vi "Highlight Selected Row in Table Control 2012 NIVerified.vi"() -> ()   [LabVIEW 2012]
doc: "This example lets you highlight a row based on which row a user clicks on. It changes the background color and then changes it back to blank when another row is clicked on."
panel:
  in  "stop":bool
  in  "Table Control":string[][](table)
  # "Overview: This example demonstrates a common practice of dealing with Tables programmatically,which lets you highlight a row based on which row a user clicks on. \nRequirements: LabVIEW 2012 (or compatible)\nInstruction:\n1. Run the VI\n2. Click on a row to highlight it."
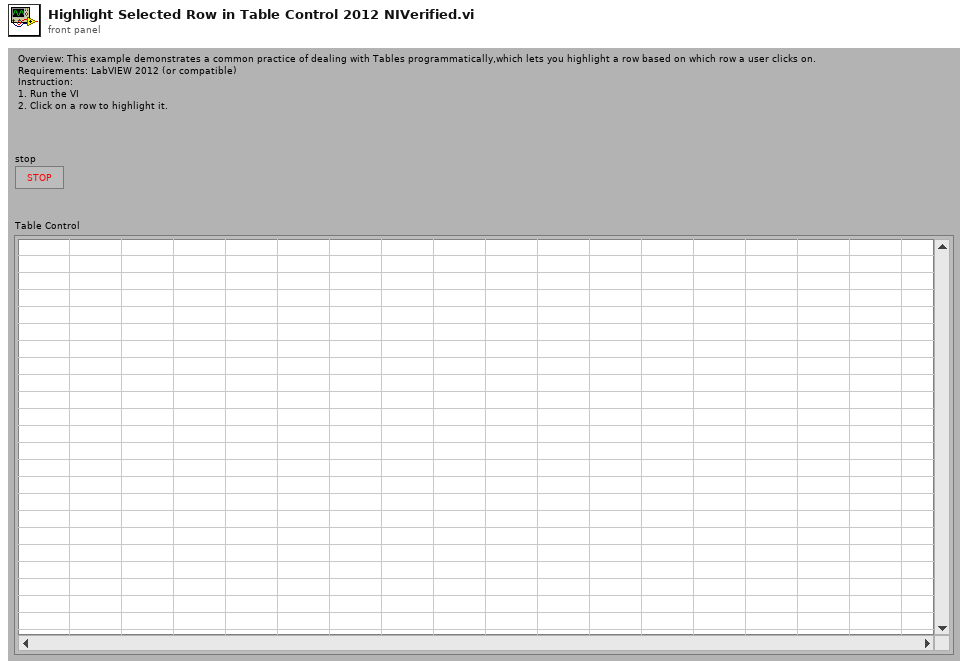
[diagram p1: front panel]
types:
  T1 = typedef "LVRowAndColumnTypeDef.ctl" = cluster{"Row":i32, "Column":i32}
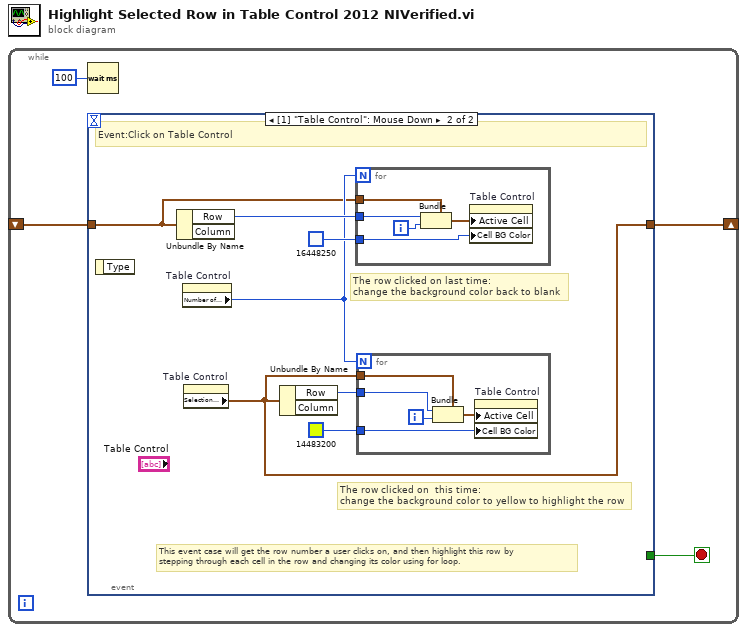
[diagram p0: block diagram]
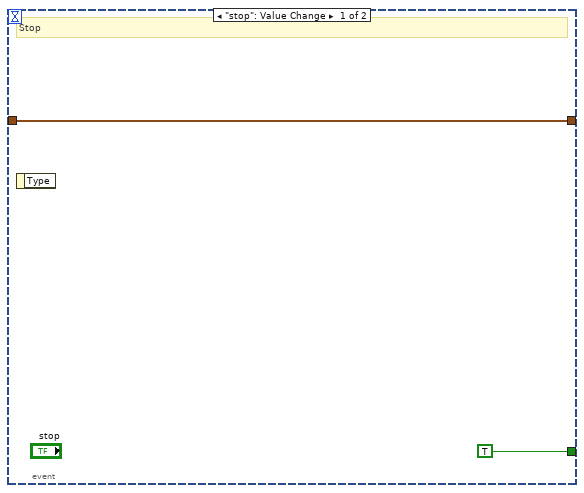
[diagram p2: hidden frame]
diagram:
  n1 = while {
    shift-right: [w3] -> _
    shift-left: _ -> [w2]
    stop <- w1 stop-if-true
    n2 = Wait (ms)(milliseconds to wait=u32 100) -> ()  [unwired: 1 out]
    n3 = event shown="[1] \"Table Control\": Mouse Down" {
      selector: _ -> [_ _]
      dyn-events: _ -> [_ _]
      timeout: _ -> [_ _]
      tunnel: [w6 w7] -> w3
      tunnel: w2 -> [w6 w8]
      tunnel: [TRUE _] -> w1
      event "stop": Value Change {
        # "Stop"
        n4 = event-data() -> ()  [unwired: 1 in, 1 out]
      }
      event "Table Control": Mouse Down {
        # "This event case will get the row number a user clicks on, and then highlight this row by \nstepping through each cell in the row and changing its color using for loop."
        # "The row clicked on  this time:\nchange the background color to yellow to highlight the row"
        # "The row clicked on last time:\nchange the background color back to blank"
        # "Event:Click on Table Control"
        n5 = event-data() -> ()  [unwired: 1 in, 1 out]
        n6 = Unbundle By Name(w8) -> ("Row"=w11:i32)  [unwired: 1 out]
        n7 = property on="Table Control" class="Tbl (strict)"() -> ("Number of Columns"=w9:u32)  [unwired: 2 in, 2 out]
        n8 = property on="Table Control" class="Tbl (strict)"() -> ("Selection Start"=w7:T1)  [unwired: 2 in, 2 out]
        n9 = Unbundle By Name(w7) -> ("Row"=w12:i32)  [unwired: 1 out]
        n10 = for {
          N: w9 -> [_]
          tunnel: u32 16448250 -> [w18]
          tunnel: w8 -> [w17]
          tunnel: w11 -> [w16]
          i -> [w15]
          n11 = Bundle(cluster=w17, "Row"=w16, "Column"=w15) -> (w14:T1)
          n12 = property on="Table Control" class="Tbl (strict)"("Active Cell"=w14, "Cell BG Color"=w18) -> ()  [unwired: 2 in, 2 out]
        }
        n13 = for {
          N: w9 -> [_]
          tunnel: u32 14483200 -> [w23]
          tunnel: w7 -> [w22]
          tunnel: w12 -> [w21]
          i -> [w20]
          n14 = Bundle(cluster=w22, "Row"=w21, "Column"=w20) -> (w19:T1)
          n15 = property on="Table Control" class="Tbl (strict)"("Active Cell"=w19, "Cell BG Color"=w23) -> ()  [unwired: 2 in, 2 out]
        }
      }
    }
  }
